vi "ImageResample.vi"(1 "image buffer in":T1, 2 "Yresolution":i32=50, 3 "Xresolution":i32=50, 4 "imagein":T1) -> (0 "Image Out":T1)   [LabVIEW 2018]
uses:
  <vilib>/vision/Image Controls.llb/IMAQ Image.ctl
panel:
  out "数组 2":dbl[](array[numeric])
  out "数组":dbl[](array[numeric])
  out "Y Resolution 2":i32
  out "X Resolution 2":i32
  out "Y Resolution":i32
  out "X Resolution":i32
  out "Image 2":T1(plugin-control)
  out "Image":T1(plugin-control)
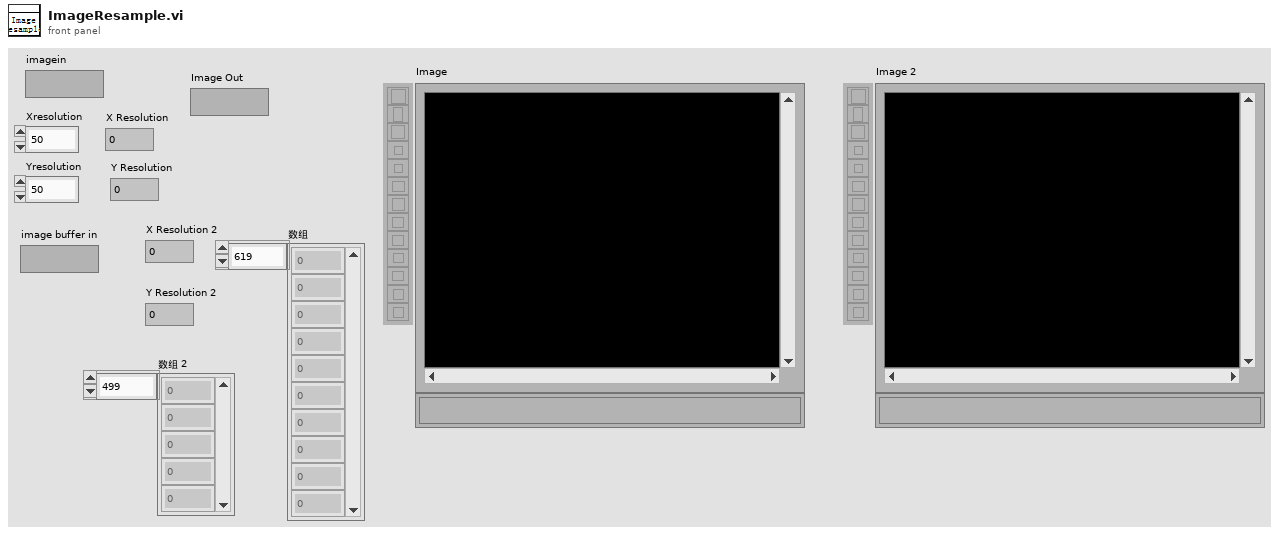
[diagram p1: front panel]
types:
  T1 = typedef "IMAQ Image.ctl" = refnum<image>
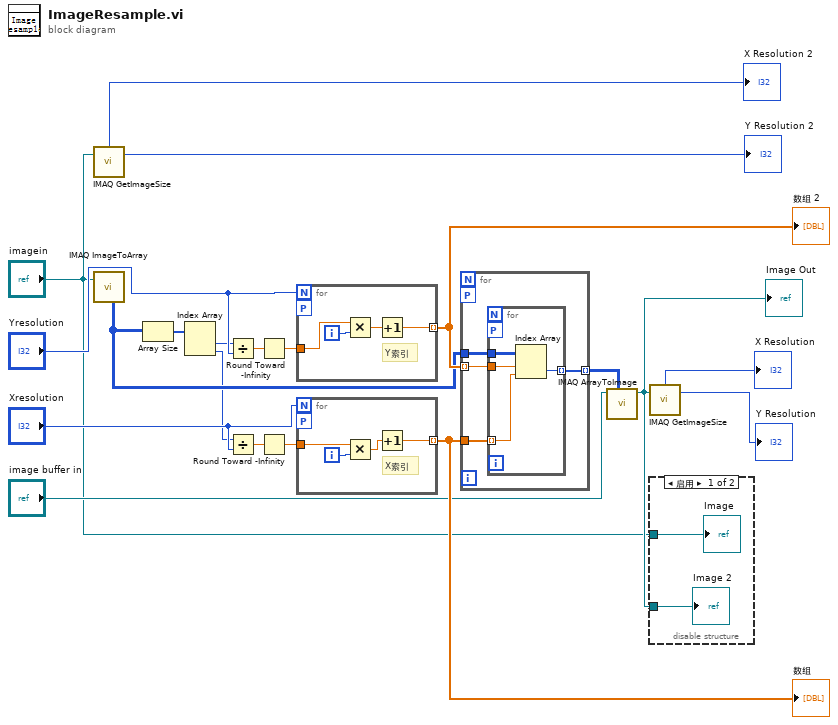
[diagram p0: block diagram]
diagram:
  n1 = call "IMAQ GetImageSize"("Image"="imagein") -> ("Y Resolution"=→"Y Resolution 2":i32, "X Resolution"=→"X Resolution 2":i32)  [unwired: 3 in, 1 out]
  n2 = call "IMAQ ImageToArray"("Image"="imagein") -> ("Image Pixels (U16)"=w3:u16[][])  [unwired: 3 in, 4 out]
  n3 = Array Size(array=w3) -> (size(s)=w20:i32[])
  n4 = Index Array(array=w20) -> (element #1=w2:i32, element #2=w1:i32)  [unwired: 2 in]
  n5 = Divide(x=w2, y="Yresolution") -> (x/y=w17:dbl)
  n6 = Divide(x=w1, y="Xresolution") -> (x/y=w19:dbl)
  n7 = Round Toward -Infinity(1:w17) -> (0:w16:dbl)
  n8 = Round Toward -Infinity(1:w19) -> (0:w15:dbl)
  n9 = for "For循环" {
    N: "Yresolution" -> [_]
    tunnel: w16 -> [w24]
    tunnel: [w21] -> w12 mode=indexing
    workers-P: _ -> [_]
    i -> [w23]
    # "Y索引"
    n10 = Multiply(x=w24, y=w23) -> (x*y=w22:dbl)
    n11 = Increment(x=w22) -> (x+1=w21:dbl)
  }
  "数组 2" <- w12
  n12 = for "For循环" {
    N: "Xresolution" -> [_]
    tunnel: w15 -> [w28]
    tunnel: [w25] -> w13 mode=indexing
    workers-P: _ -> [_]
    i -> [w27]
    # "X索引"
    n13 = Multiply(x=w28, y=w27) -> (x*y=w26:dbl)
    n14 = Increment(x=w26) -> (x+1=w25:dbl)
  }
  "数组" <- w13
  n15 = for "For循环" {
    tunnel: w13 -> [w31]
    tunnel: w12 -> [w32] mode=indexing
    tunnel: w3 -> [w30]
    tunnel: [w29] -> w10 mode=indexing
    workers-P: _ -> [_]
    n16 = for "For循环" {
      tunnel: w32 -> [w33]
      tunnel: w31 -> [w34] mode=indexing
      tunnel: w30 -> [w36]
      tunnel: [w35] -> w29 mode=indexing
      workers-P: _ -> [_]
      n17 = Index Array(array=w36, index (row)=w33, index (col)=w34) -> (element=w35:u16)
    }
  }
  n18 = call "IMAQ ArrayToImage"("Image Pixels (U16)"=w10, "Image"="image buffer in") -> ("Image Out"=w9:T1)  [unwired: 8 in, 1 out]
  "Image Out" <- w9
  n19 = call "IMAQ GetImageSize"("Image"=w9) -> ("Y Resolution"=→"Y Resolution":i32, "X Resolution"=→"X Resolution":i32)  [unwired: 3 in, 1 out]
  n20 = disable-structure shown="启用" {
    disable-tunnel: "imagein" -> [w38 _]
    disable-tunnel: w9 -> [w37 _]
    frame Enabled {
      "Image" <- w38
      "Image 2" <- w37
    }
    frame Disabled {
    }
  }
